vi "Drive Controller.vi"(8 "error in":errorcluster) -> ()   [LabVIEW 2016]
doc: "This VI executes continuously carrying out the current operation and responding to updates or new operation requests. It will often contain the timing or control code that is difficult to place directly in TeleOp. This VI generally opens all sensors and motors and isolates the rest of the robot code from knowing implementation details of how the operations are carried out."
uses:
  Drive Setpoints.ctl
  Drive Operations.ctl
  <vilib>/Rock Robotics/WPI/SafetyOutput/WPI_SafetyOutputConfigMenu.ctl
  <vilib>/Rock Robotics/SystemInterfaces/DIO/FPGA_DIOPWMChannel.ctl
  <vilib>/Rock Robotics/SystemInterfaces/DIO/FPGA_DIOChannel.ctl
  <vilib>/Rock Robotics/WPI/RobotDrive/WPI_RobotDriveOpen4MotorWithJaguar.vi
  <vilib>/Rock Robotics/WPI/Counter/WPI_CounterDigitalInputToDigitalSource.vi
  <vilib>/Rock Robotics/WPI/Gyro/WPI_GyroAnalogOpen.vi
panel:
  out "Setpoints":T1(graph)
  out "Current\nCmd":string
  # "Tip: It may be helpful to observe inputs and sensor values.\nYou may also want to display tuning or debugging controls."
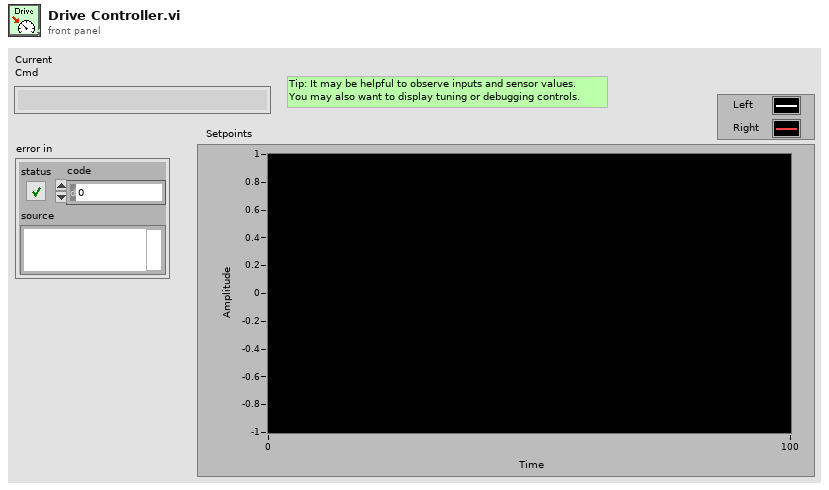
[diagram p1: front panel]
types:
  T1 = cluster{"Left Setpoint":dbl, "Right Setpoint":dbl}
  T2 = typedef "FPGA_DIOChannel.ctl" = enum8{"DIO 0", "DIO 1", "DIO 2", "DIO 3", "DIO 4", "DIO 5", "DIO 6", "DIO 7", "DIO 8", "DIO 9", "DIO MXP 0", "DIO MXP 1", "DIO MXP 2", "DIO MXP 3", "DIO MXP 4", "DIO MXP 5", "DIO MXP 6", "DIO MXP 7", "DIO MXP 8", "DIO MXP 9", "DIO MXP 10", "DIO MXP 11", "DIO MXP 12", "DIO MXP 13", "DIO MXP 14", "DIO MXP 15", "SPI Port CS1", "SPI Port CS2", "SPI Port CS3", "SPI Port MISO", "SPI Port MOSI", "Invalid"}
  T3 = typedef "FPGA_DIOPWMChannel.ctl" = enum8{"PWM 0", "PWM 1", "PWM 2", "PWM 3", "PWM 4", "PWM 5", "PWM 6", "PWM 7", "PWM 8", "PWM 9", "PWM MXP 0", "PWM MXP 1", "PWM MXP 2", "PWM MXP 3", "PWM MXP 4", "PWM MXP 5", "PWM MXP 6", "PWM MXP 7", "PWM MXP 8", "PWM MXP 9", "Invalid"}
  T4 = typedef "WPI_SafetyOutputConfigMenu.ctl" = enum16{"Enable", "Disable"}
  T5 = typedef "Drive Setpoints.ctl" = cluster{"Operation":T6, "Left Setpoint":dbl, "Right Setpoint":dbl, "Duration":dbl, "Distance":dbl, "Angle":dbl}
  T6 = typedef "Drive Operations.ctl" = enum16{"Reserve", "Read Current", "Immediate", "Drive for Time", "Drive for Distance", "Drive For Angle"}
  T7 = typedef "WPI_RobotDriveDevRef.ctl" = cluster{"DevStatus":errorcluster, "Motors[]":T8[], "Square Inputs":bool, "Max Output":dbl}
  T8 = typedef "WPI_MotorControlDeviceRef.ctl" = cluster{"DeviceStatus":errorcluster, "Type":T9, "PWM":cluster{"PWM Channel":T3, "DeadBand":T10}, "CAN":cluster{"Device Number":u8, "SetOutput VI Ref":variant, "GetOutput VI Ref":variant, "Enable VI Ref":variant, "Disable VI Ref":variant, "Data":variant}, "Invert":bool}
  T9 = typedef "WPI_MotorControlType.ctl" = enum16{"PWM", "CAN"}
  T10 = typedef "WPI_PWMDeadband.ctl" = cluster{"Name":string, "maxPositivePwm":i32, "minPositivePwm":i32, "centerPwm":i32, "maxNegativePwm":i32, "minNegativePwm":i32, "angularRange":u16}
  T11 = typedef "WPI_DigitalInputDevRef.ctl" = cluster{"DevStatus":errorcluster, "DIO Channel":T2}
  T12 = typedef "FPGA_CounterEncoderSourceConvertionLVSourceType.ctl" = cluster{"DevStatus":errorcluster, "AnalogTriggerMode?":bool, "DigitalMode":cluster{"DIO Channel":T13}, "AnalogTriggerMode":cluster{"AnalogTriggerIndex":T14, "OutputType":T15}}
  T13 = typedef "FPGA_DIODigitalSourceChannel.ctl" = enum8{"DIO 0", "DIO 1", "DIO 2", "DIO 3", "DIO 4", "DIO 5", "DIO 6", "DIO 7", "DIO 8", "DIO 9", "DIO MXP 0", "DIO MXP 1", "DIO MXP 2", "DIO MXP 3", "DIO MXP 4", "DIO MXP 5", "DIO MXP 6", "DIO MXP 7", "DIO MXP 8", "DIO MXP 9", "DIO MXP 10", "DIO MXP 11", "DIO MXP 12", "DIO MXP 13", "DIO MXP 14", "DIO MXP 15", "Disabled"}
  T14 = typedef "FPGA_AnalogTriggerIndex.ctl" = enum8{"Trig 0", "Trig 1", "Trig 2", "Trig 3", "Trig 4", "Trig 5", "Trig 6", "Trig 7", "Invalid"}
  T15 = typedef "FPGA_AnalogTriggerOutType.ctl" = enum16{"InWindow", "TriggerState", "Rising", "Falling"}
  T16 = typedef "WPI_GyroDevRef.ctl" = cluster{"DevStatus":errorcluster, "Analog Channel":T17, "Offset":dbl, "Gain (VoltsPerDegree/Second)":dbl, "Gyro Type":enum16{"Analog", "XRS450"}, "Handle":i32, "SPI Bus":T18, "Device Found":bool, "Sample Rate":dbl, "Calibrate On Open":bool}
  T17 = typedef "FPGA_AIChannel.ctl" = enum8{"AI 0", "AI 1", "AI 2", "AI 3", "AI MXP 0", "AI MXP 1", "AI MXP 2", "AI MXP 3", "Invalid"}
  T18 = typedef "spi_bus.ctl" = enum16{"SPI On-Board, CS0", "SPI On-Board, CS1", "SPI On-Board, CS2", "SPI On-Board, CS3", "SPI MXP", "Invalid"}
  T19 = typedef "WPI_EncoderDevRef.ctl" = cluster{"DevStatus":errorcluster, "EncoderIndex":T20, "CounterIndex":T21, "DistancePerCount":dbl, "Decoding Type":T22}
  T20 = typedef "FPGA_EncoderIdx.ctl" = enum8{"Enc 0", "Enc 1", "Enc 2", "Enc 3", "Enc 4", "Enc 5", "Enc 6", "Enc 7", "Invalid"}
  T21 = typedef "FPGA_CounterCtrSystemIndex.ctl" = enum8{"Ctr 0", "Ctr 1", "Ctr 2", "Ctr 3", "Ctr 4", "Ctr 5", "Ctr 6", "Ctr 7", "Invalid"}
  T22 = typedef "WPI_EncoderType.ctl" = enum16{"1x", "2x", "4x"}
  T23 = typedef "Command Status Info.ctl" = cluster{"Name":string, "Status":T24, "notifier out":T25}
  T24 = typedef "Completion Status.ctl" = enum16{"Successful", "Aborted", "Incomplete"}
  T25 = typedef "Completion Notifier.ctl" = refnum<notifier>
  T26 = cluster{"SubSystem Data":T5, cluster{"Start Time (ms)":u32, "Iterations":i32}, cluster{"Command Info":T23, "Description":string, "SubSystem Data":T5, "notifier out":refnum<notifier>, "Subsystem Name":string}}
  T27 = cluster{"SubSystem Data":T5, cluster{"Start Time (ms)":u32, "Iterations":i32}, "Default Command Arguments":cluster{"Command Info":T23, "Description":string, "SubSystem Data":T5, "notifier out":refnum<notifier>, "Subsystem Name":string}}
  T28 = cluster{"Left Setpoint (UI)":dbl, "Right Setpoint (UI)":dbl}
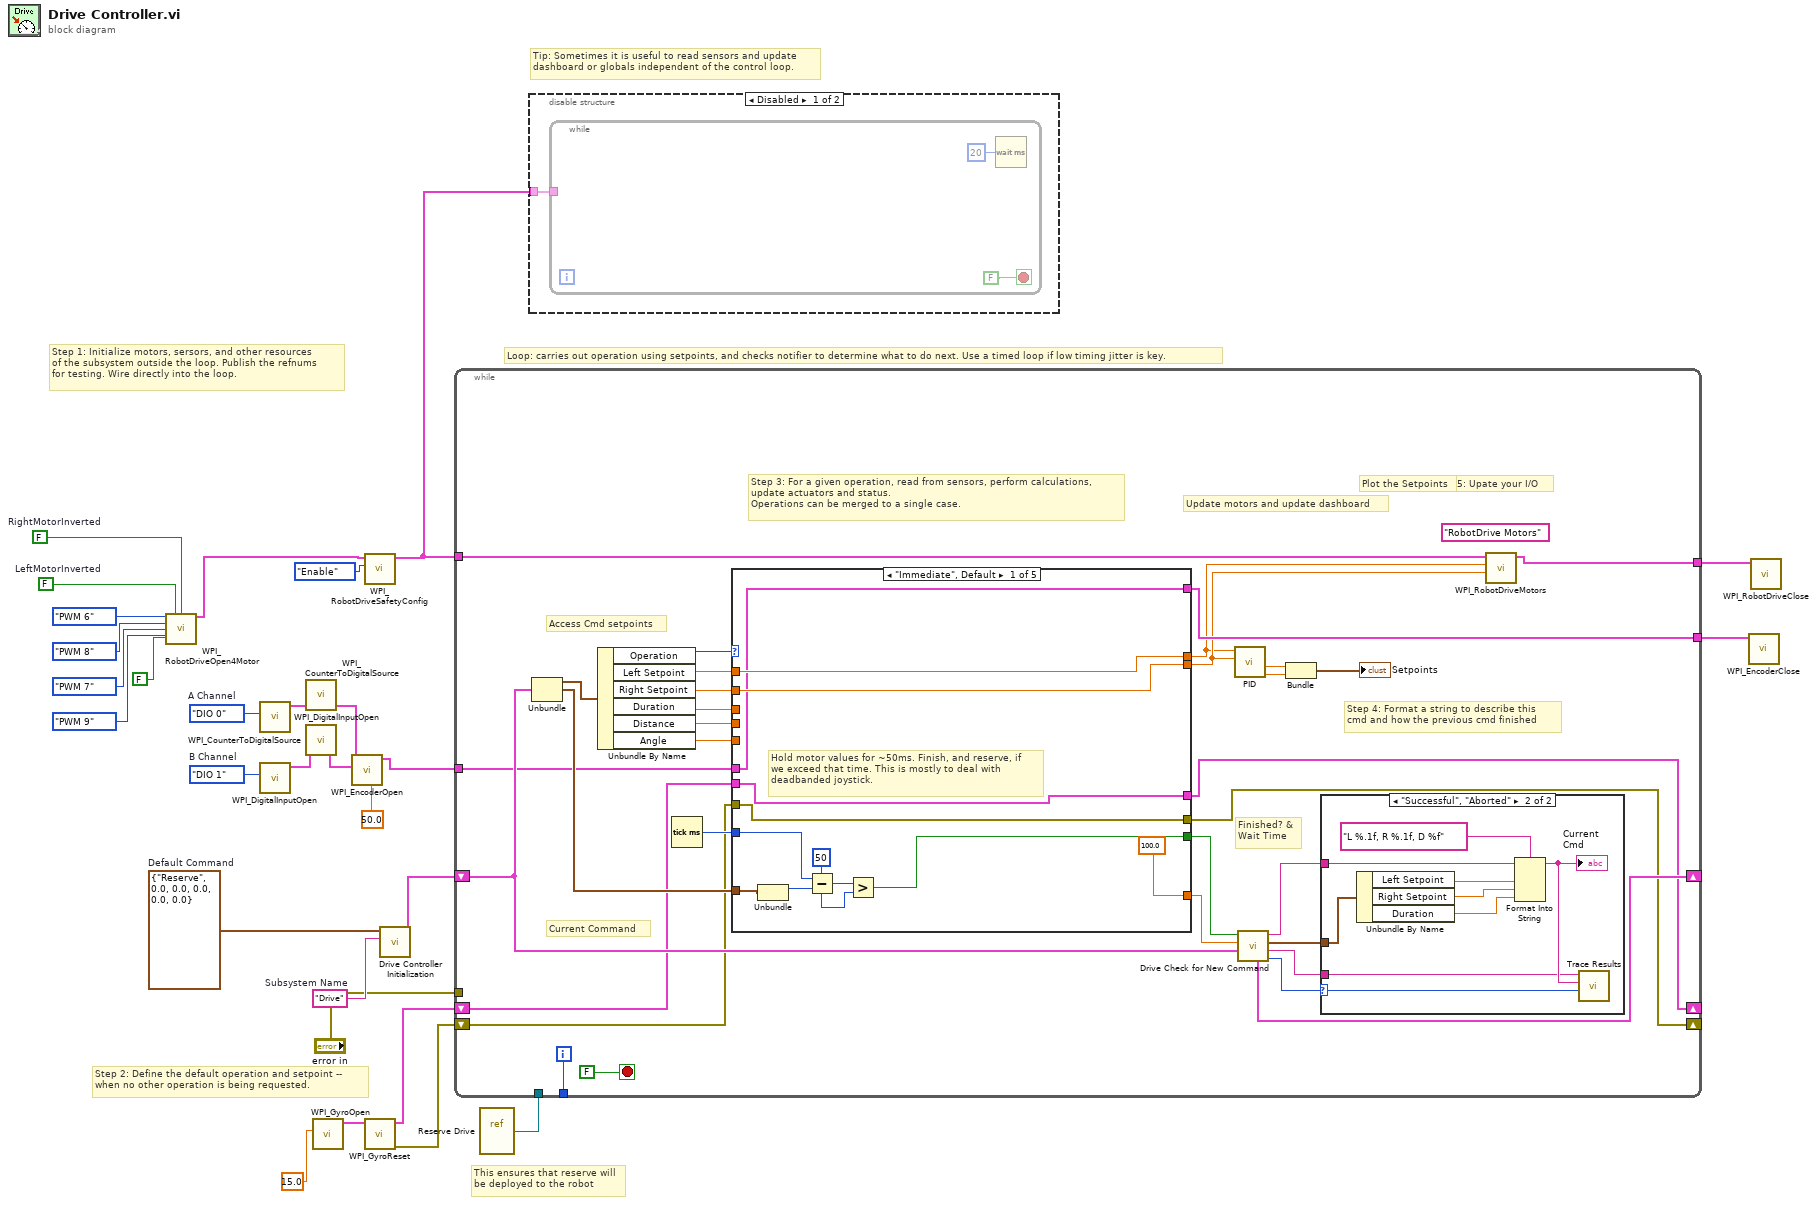
[diagram p0: block diagram]
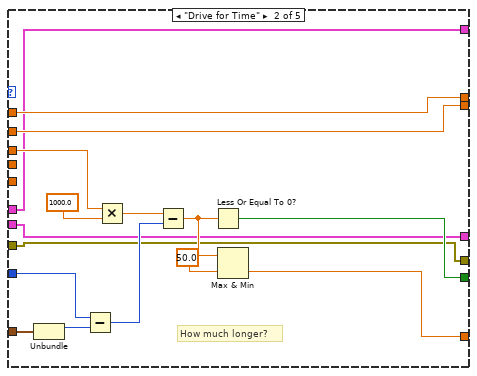
[diagram p4: hidden frame]
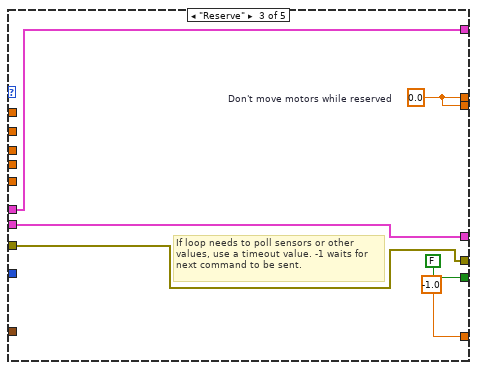
[diagram p5: hidden frame]
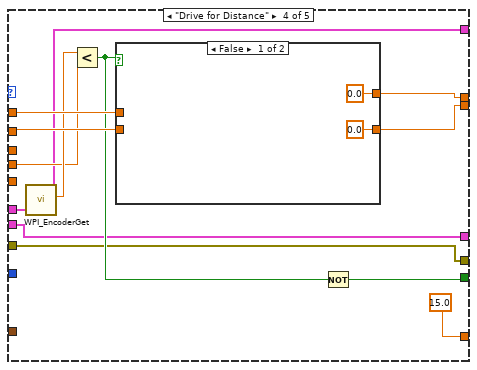
[diagram p6: hidden frame]
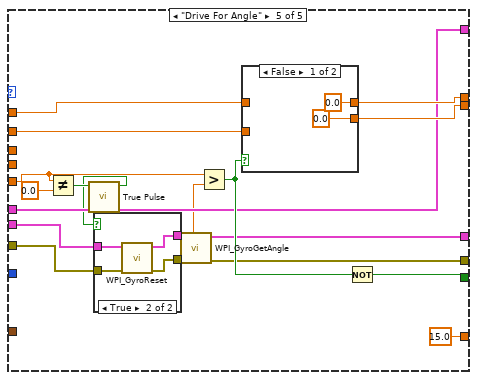
[diagram p8: hidden frame]
diagram:
  w14 = FPGA_DIOChannel."DIO 1"  # B Channel
  w13 = FPGA_DIOChannel."DIO 0"  # A Channel
  w26 = FALSE  # LeftMotorInverted
  w27 = FALSE  # RightMotorInverted
  w28 = T5 {"Operation"=enum."Reserve", "Left Setpoint"=0.0, "Right Setpoint"=0.0, "Duration"=0.0, "Distance"=0.0, "Angle"=0.0}  # Default Command
  w29 = "Drive"  # Subsystem Name
  # "This ensures that reserve will\nbe deployed to the robot"
  # "Tip: Sometimes it is useful to read sensors and update\ndashboard or globals independent of the control loop."
  # "Step 2: Define the default operation and setpoint --\nwhen no other operation is being requested."
  # "Step 1: Initialize motors, sersors, and other resources\nof the subsystem outside the loop. Publish the refnums\nfor testing. Wire directly into the loop."
  # "Loop: carries out operation using setpoints, and checks notifier to determine what to do next. Use a timed loop if low timing jitter is key."
  n1 = call-poly <vilib>:"WPI_RobotDriveOpen4Motor.vi"("Rear Left Motor"=FPGA_DIOPWMChannel."PWM 6", "Rear Left Motor Inverted"=w26, "Rear Right Motor Inverted"=w27, "Rear Right Motor"=FPGA_DIOPWMChannel."PWM 8", "Front Left Motor"=FPGA_DIOPWMChannel."PWM 7", "Front Right Motor"=FPGA_DIOPWMChannel."PWM 9", "Front Right Motor Inverted"=FALSE) -> ("RobotDriveDevRef"=w25:T7)  [unwired: 7 in, 1 out]
  n2 = call <vilib>:"WPI_DigitalInputOpen.vi"("DIO Channel"=w13) -> ("DigitalInputDevRef"=w10:T11)  [unwired: 1 in, 9 out]
  n3 = call <vilib>:"WPI_DigitalInputOpen.vi"("DIO Channel"=w14) -> ("DigitalInputDevRef"=w11:T11)  [unwired: 1 in, 9 out]
  n4 = call-poly <vilib>:"WPI_CounterToDigitalSource.vi"("DigitalInputDevRef"=w10) -> ("Digital Source"=w9:T12)  [unwired: 6 out]
  n5 = call-poly <vilib>:"WPI_CounterToDigitalSource.vi"("DigitalInputDevRef"=w11) -> ("Digital Source"=w12:T12)  [unwired: 6 out]
  n6 = call-poly <vilib>:"WPI_GyroOpen.vi"("Analog Channel"=15.0 ("Sample Rate (ms)")) -> ("GyroDevRef"=w4:T16)  [unwired: 8 in, 2 out]
  n7 = call <vilib>:"WPI_EncoderOpen.vi"("DistancePerCount"=50.0, "BSource"=w12, "ASource"=w9) -> ("EncoderDevRef"=w7:T19)  [unwired: 5 in, 3 out]
  n8 = call <vilib>:"WPI_RobotDriveSafetyConfig.vi"("mode"=WPI_SafetyOutputConfigMenu."Enable", "RobotDriveDevRef"=w25) -> ("RobotDriveDevRef"=w23:T7)  [unwired: 8 in, 1 out]
  n9 = call <vilib>:"WPI_GyroReset.vi"("GyroDevRef"=w4) -> ("error out"=w1:errorcluster, "GyroDevRef"=w2:T16)  [unwired: 9 in]
  n10 = call "Drive Controller Initialization.vi"("Subsystem Name"=w29, "Default Command"=w28) -> ("output cluster"=w21:T26)  [unwired: 9 in]
  n11 = vi-ref "Reserve Drive.vi"() -> (w20:refnum<vi>)
  n12 = while {
    shift-right: [w51] -> _
    shift-left: w21 -> [w44]
    tunnel: [w60] -> _
    tunnel: w23 -> [w58]
    tunnel: "error in" -> [_]
    tunnel: w20 -> [_]
    tunnel: w7 -> [w42]
    tunnel: [w39] -> w6
    tunnel: [w38] -> w5
    shift-right: [w34] -> _
    shift-left: w1 -> [w37]
    shift-right: [w35] -> _
    shift-left: w2 -> [w36]
    i -> [w60]
    stop <- FALSE stop-if-true
    (unwired) "RobotDrive Motors" ("Name")
    # "Step 5: Upate your I/O"
    # "Step 4: Format a string to describe this\ncmd and how the previous cmd finished"
    # "Current Command"
    # "Update motors and update dashboard"
    # "Plot the Setpoints"
    # "Access Cmd setpoints"
    # "Finished? &\nWait Time"
    # "Step 3: For a given operation, read from sensors, perform calculations,\nupdate actuators and status.\nOperations can be merged to a single case."
    n13 = Unbundle(w44) -> ("SubSystem Data"=w57:T5, w45:cluster{"Start Time (ms)":u32, "Iterations":i32})  [unwired: 1 out]
    n14 = Unbundle By Name(w57) -> ("Operation"=w56:T6, "Left Setpoint"=w55:dbl, "Right Setpoint"=w54:dbl, "Duration"=w53:dbl, "Distance"=w43:dbl, "Angle"=w40:dbl)
    n15 = Tick Count (ms)() -> (millisecond timer value=w41:u32)
    n16 = case shown="\"Immediate\", Default" w56 {
      tunnel: [100.0 w86 -1.0 15.0 15.0] -> w50
      tunnel: [w75 w93 FALSE ("ignore previous (F)") w108 w134] -> w49
      tunnel: w45 -> [w74 w95 _ _ _]
      tunnel: [w81 w92 w102 w115 w140] -> w32
      tunnel: [w80 w91 w102 w114 w137] -> w33
      tunnel: w55 -> [w81 w92 _ w116 w139]
      tunnel: w54 -> [w80 w91 _ w113 w138]
      tunnel: w53 -> [_ w90 _ _ _]
      tunnel: w43 -> [_ _ _ w111 _]
      tunnel: w42 -> [w73 w85 w101 w117 w133]
      tunnel: w41 -> [w76 w89 _ _ _]
      tunnel: w40 -> [_ _ _ _ w125]
      tunnel: [w73 w85 w101 w107 w133] -> w38
      tunnel: w37 -> [w71 w83 w99 w105 w128]
      tunnel: w36 -> [w72 w84 w100 w106 w129]
      tunnel: [w72 w84 w100 w106 w127] -> w35
      tunnel: [w71 w83 w99 w105 w126] -> w34
      frame "Immediate", Default {
        # "Hold motor values for ~50ms. Finish, and reserve, if\nwe exceed that time. This is mostly to deal with\ndeadbanded joystick."
        n17 = Unbundle(w74) -> ("Start Time (ms)"=w77:u32)  [unwired: 1 out]
        n18 = Subtract(x=w76, y=w77) -> (x-y=w78:u32)
        n19 = Greater?(x=w78, y=u8 50 ("Left Motor")) -> (0:w75:bool)
      }
      frame "Drive for Time" {
        # "How much longer?"
        n20 = Unbundle(w95) -> ("Start Time (ms)"=w94:u32)  [unwired: 1 out]
        n21 = Subtract(x=w89, y=w94) -> (x-y=w98:u32)
        n22 = Multiply(x=w90, y=1000.0) -> (x*y=w97:dbl)
        n23 = Subtract(x=w97, y=w98) -> (x-y=w88:dbl)
        n24 = Less Or Equal To 0?(x=w88) -> (x <= 0?=w93:bool)
        n25 = Max & Min(x=w88, y=50.0) -> (min(x,y)=w86:dbl)  [unwired: 1 out]
      }
      frame "Reserve" {
        w102 = 0.0  # Don't move motors while reserved
        # "If loop needs to poll sensors or other\nvalues, use a timeout value. -1 waits for\nnext command to be sent."
      }
      frame "Drive for Distance" {
        n26 = call <vilib>:"WPI_EncoderGet.vi"("EncoderDevRef"=w117) -> ("Distance"=w112:dbl, "EncoderDevRef"=w107:T19)  [unwired: 5 in, 4 out]
        n27 = Less?(x=w112, y=w111) -> (x < y?=w109:bool)
        n28 = case shown="False" w109 {
          tunnel: [0.0 ("Left Setpoint") w121] -> w115
          tunnel: w116 -> [_ w121]
          tunnel: w113 -> [_ w120]
          tunnel: [0.0 ("Right Setpoint") w120] -> w114
          frame False {
          }
          frame True {
          }
        }
        n29 = Not(x=w109) -> (.not. x?=w108:bool)
      }
      frame "Drive For Angle" {
        n30 = Not Equal?(x=w125, y=0.0) -> (x != y?=w123:bool)
        n31 = call "True Pulse.vi"("y"=w123) -> (".not. (x .or. y)?"=w122:bool)  [unwired: 10 in]
        n32 = case shown="True" w122 {
          tunnel: [w142 w146] -> w131
          tunnel: [w141 w145] -> w130
          tunnel: w129 -> [w142 w144]
          tunnel: w128 -> [w141 w143]
          frame False {
          }
          frame True {
            n33 = call <vilib>:"WPI_GyroReset.vi"("error in"=w143, "GyroDevRef"=w144) -> ("error out"=w145:errorcluster, "GyroDevRef"=w146:T16)  [unwired: 8 in]
          }
        }
        n34 = call <vilib>:"WPI_GyroGetAngle.vi"("error in"=w130, "GyroDevRef"=w131) -> ("error out"=w126:errorcluster, "Angle"=w132:dbl, "GyroDevRef"=w127:T16)  [unwired: 5 in, 2 out]
        n35 = Greater?(x=w125, y=w132) -> (0:w135:bool)
        n36 = case shown="False" w135 {
          tunnel: [0.0 ("Left Setpoint") w150] -> w140
          tunnel: w139 -> [_ w150]
          tunnel: w138 -> [_ w149]
          tunnel: [0.0 ("Right Setpoint") w149] -> w137
          frame False {
          }
          frame True {
          }
        }
        n37 = Not(x=w135) -> (.not. x?=w134:bool)
      }
    }
    n38 = call "PID.vi"("Right Setpoint"=w33, "Left Setpoint"=w32) -> ("Right Setpoint (UI)"=w30:dbl, "Left Setpoint (UI)"=w31:dbl)  [unwired: 6 in, 2 out]
    n39 = call "Drive Check for New Command.vi"("input cluster"=w44, "Wait time (ms)"=w50, "Finished?"=w49) -> ("Completion"=w52:T24, "Subsystem Name"=w46:string, "SetPoint"=w47:T5, "Initial Trace String"=w48:string, "output cluster"=w51:T27)  [unwired: 4 in]
    n40 = Bundle("Left Setpoint (UI)"=w31, "Right Setpoint (UI)"=w30) -> (→"Setpoints":T28)  [unwired: 1 in]
    n41 = case shown="\"Successful\", \"Aborted\"" w52 {
      selector: w52 -> [_ w70]
      tunnel: w48 -> [_ w65]
      tunnel: w47 -> [_ w66]
      tunnel: w46 -> [_ w62]
      frame "Incomplete", Default {
        # "Continuing current command"
      }
      frame "Successful", "Aborted" {
        # "Report and setup for next command"
        n42 = Unbundle By Name(w66) -> ("Left Setpoint"=w68:dbl, "Right Setpoint"=w69:dbl, "Duration"=w63:dbl)
        n43 = Format Into String(format string="L %.1f, R %.1f, D %f", initial string=w65, w68, w69, w63) -> (resulting string=w64:string)  [unwired: 1 in, 1 out]
        "Current\nCmd" <- w64
        n44 = call <vilib>:"Trace Results.vi"("Status of previous command"=w70, "Description"=w64, "Subsystem"=w62) -> ()  [unwired: 9 in]
      }
    }
    n45 = call <vilib>:"WPI_RobotDriveMotors.vi"("RightSpeed"=w33, "LeftSpeed"=w32, "RobotDriveDevRef"=w58) -> ("RobotDriveDevRef"=w39:T7)  [unwired: 1 in, 7 out]
  }
  n46 = disable-structure shown="Disabled" {
    disable-tunnel: w23 -> [w151 _]
    frame Disabled {
      n47 = while {
        tunnel: w151 -> [_]
        stop <- FALSE stop-if-true
        n48 = Wait (ms)(milliseconds to wait=u32 20) -> ()  [unwired: 1 out]
      }
    }
    frame Enabled {
    }
  }
  n49 = call <vilib>:"WPI_EncoderClose.vi"("EncoderDevRef"=w5) -> ()  [unwired: 10 in, 1 out]
  n50 = call <vilib>:"WPI_RobotDriveClose.vi"("RobotDriveDevRef"=w6) -> ()  [unwired: 10 in, 1 out]
